vi "dIMU_Accel_gs.vi"(7 "Port":T1 items=["Port 1", "Port 2", "Port 3", "Port 4"], 8 "Calibrate":bool, 9 "Maximum Range":enum8{"2g", "4g", "8g"}(ring), 10 "Calibrate Axis":enum8{"Z", "X", "Y"}(ring), 11 "NXT":T2) -> (0 "Z Accel (g)":dbl, 1 "Y Accel (g)":dbl, 2 "X Accel (g)":dbl, 3 "NXT":T2)   [LabVIEW 2010]
uses:
  <vilib>/NXT/Subs/LVHSConnector.ctl
  <vilib>/NXT/Block Support/NXT_InputPort.ctl
  <vilib>/NXT/Block Support/HWPage.SensorType.ctl
  <vilib>/NXT/Block Support/HWPage.SensorMode.ctl
  <vilib>/NXT/Dual Mode Library/Sensors/i2c_sensors.vi
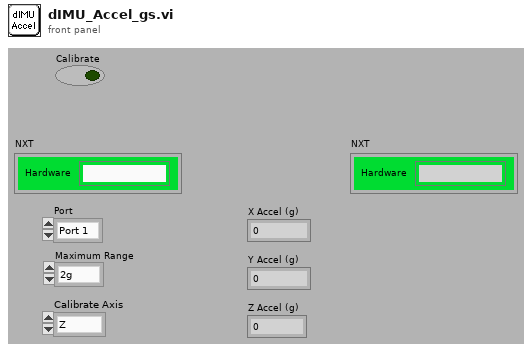
[diagram p1: front panel]
types:
  T1 = typedef "NXT_InputPort.ctl" = u8
  T2 = typedef "LVHSConnector.ctl" = cluster{"Hardware":string, "Flattened String":string}
  T3 = typedef "HWPage.SensorType.ctl" = u8
  T4 = typedef "HWPage.SensorMode.ctl" = u8
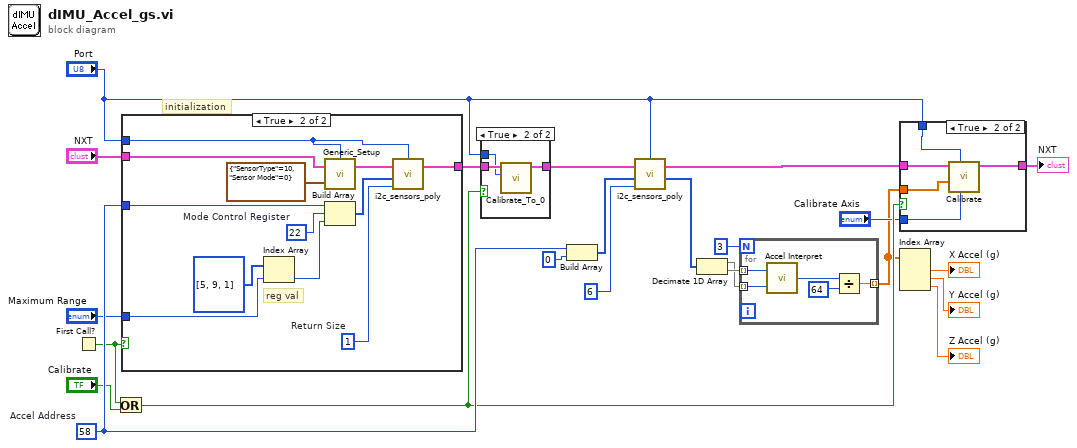
[diagram p0: block diagram]
diagram:
  w21 = u8 58  # Accel Address
  # "initialization"
  n1 = First Call?() -> (First Call?: T/F=w11:bool)
  n2 = Or(x=w11, y="Calibrate") -> (x .or. y?=w9:bool)
  n3 = case shown="True" w11 {
    tunnel: "Maximum Range" -> [_ w35]
    tunnel: "NXT" -> [w24 w34]
    tunnel: [w24 w28] -> w13
    tunnel: "Port" -> [_ w27]
    tunnel: w21 -> [_ w26]
    frame False {
    }
    frame True {
      w29 = u8 1  # Return Size
      w32 = u8 22  # Mode Control Register
      # "reg val"
      n4 = Index Array(array=u8[] [5, 9, 1], index=w35) -> (element=w31:u8)
      n5 = call <vilib>:"Generic_Setup.vi"("Sensor Setup"=cluster{"SensorType":T3, "Sensor Mode":T4} {"SensorType"=10, "Sensor Mode"=0}, "NXT"=w34, "Port"=w27) -> ("NXT"=w33:T2)  [unwired: 1 out]
      n6 = Build Array(w26, w32, w31) -> (w30:u8[])
      n7 = call-poly <vilib>:"i2c_sensors_poly.vi"("Return Length"=w29, "Bytes to Write"=w30, "NXT"=w33, "Port"=w27) -> ("NXT"=w28:T2)  [unwired: 1 in, 2 out]
    }
  }
  n8 = case shown="True" w9 {
    tunnel: w13 -> [w37 w40]
    tunnel: [w37 w39] -> w12
    tunnel: "Port" -> [_ w38]
    frame False {
    }
    frame True {
      n9 = call "Calibrate_To_0.vi"("Port"=w38, "NXT"=w40) -> ("NXT 2"=w39:T2)  [unwired: 9 in]
    }
  }
  n10 = Build Array(w21, u8 0) -> (w19:u8[])
  n11 = call-poly <vilib>:"i2c_sensors_poly.vi"("Return Length"=u8 6, "Bytes to Write"=w19, "NXT"=w12, "Port"="Port") -> ("Bytes read"=w18:u8[], "NXT"=w6:T2)  [unwired: 1 in, 1 out]
  n12 = Decimate 1D Array(w18) -> (w16:u8[], w17:u8[])
  n13 = for {
    N: 3 -> [_]
    tunnel: w17 -> [w45] mode=indexing
    tunnel: w16 -> [w44] mode=indexing
    tunnel: [w41] -> w7 mode=indexing
    n14 = call "Accel Interpret.vi"("LSB"=w44, "MSB"=w45) -> ("Value"=w42:i16)
    n15 = Divide(x=w42, y=i16 64) -> (x/y=w41:dbl)
  }
  n16 = case shown="True" w9 {
    tunnel: w6 -> [w46 w51]
    tunnel: "Port" -> [_ w47]
    tunnel: "Calibrate Axis" -> [_ w49]
    tunnel: w7 -> [_ w50]
    tunnel: [w46 w48] -> w5
    frame False {
    }
    frame True {
      n17 = call "Calibrate.vi"("Calibrate Axis"=w49, "Port"=w47, "Accel Input Array"=w50, "NXT"=w51) -> ("NXT"=w48:T2)  [unwired: 7 in]
    }
  }
  "NXT" <- w5
  n18 = Index Array(array=w7) -> (element #1=→"X Accel (g)":dbl, element #2=→"Y Accel (g)":dbl, element #3=→"Z Accel (g)":dbl)  [unwired: 3 in]
